vi "progAspicSequence2.vi"(0 "aspic1Data":u32[](array[numeric])=[2863311530, 3149642683, 3435973836, 3722304989, 4008636142, 4294967295, 10, 10, 10, 10, 10, 10, 10, 10, 10, 10, 10, 10, 10, 10, 10, 10, 10, 10, 10, 10, 10, 10, 10, 10, 10, 10] format="%07x", 1 "aspic2Data":u32[](array[numeric])=[2863311530, 3149642683, 3435973836, 3722304989, 4008636142, 4294967295, 10, 10, 10, 10, 10, 10, 10, 10, 10, 10, 10, 10, 10, 10, 10, 10, 10, 10, 10, 10, 10, 10, 10, 10, 10, 10] format="%07x", 2 "aspic3Data":u32[](array[numeric])=[0] format="%07x") -> (9 "error out":errorcluster)   [LabVIEW 2014]
panel:
  in  "aspicmessagetype":u32=21845 format="%x"
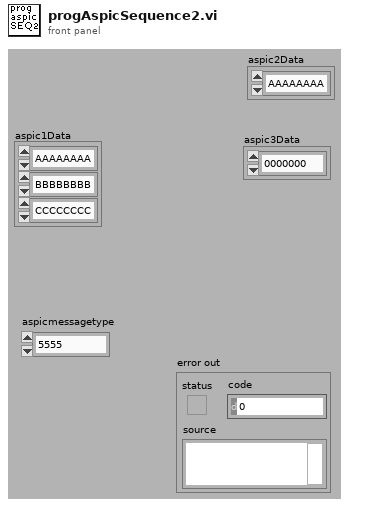
[diagram p1: front panel]
types:
  T1 = enum16{"startTSL", "writeCABAC", "readCABAC", "resetCABAC", "emissionTest", "regRead", "executeASPIC", "resetASPIC", "resetFifo18ASPIC", "resetFifo16ASPIC"}
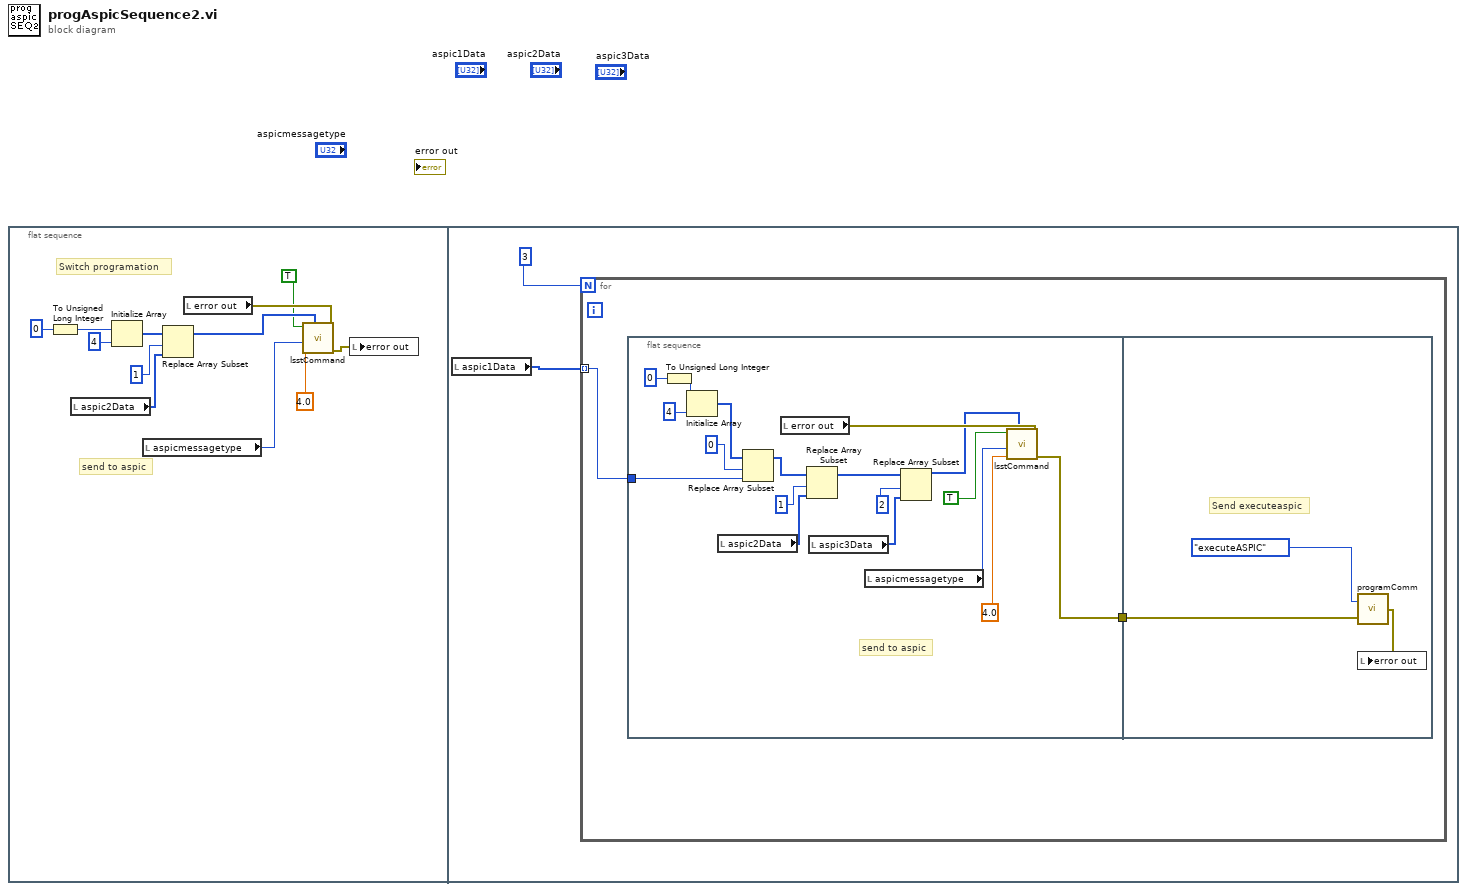
[diagram p0: block diagram]
diagram:
  n1 = flat-sequence {
    frame #0 {
      # "Switch programation"
      # "send to aspic"
      n2 = To Unsigned Long Integer(number=u32 0 ("element")) -> (unsigned 32bit integer=w9:u32)
      n3 = local read "aspic2Data"() -> (w12:u32[])
      n4 = Initialize Array(w9, 4 ("dimension size")) -> (w8:u32[])
      n5 = local read "aspicmessagetype"() -> (w5:u32)
      n6 = Replace Array Subset(array=w8, new element=w12, index=1) -> (w3:u32[])
      n7 = local read "error out"() -> (w4:errorcluster)
      n8 = call "lsstCommand.vi"("error in (no error)"=w4, "data"=w3, "nbitems"=4.0, "messagetype"=w5, "execute"=TRUE) -> ("error out"=w1:errorcluster)  [unwired: 2 in, 4 out]
      n9 = local write "error out"(w1) -> ()
    }
    frame #1 {
      n10 = local read "aspic1Data"() -> (w13:u32[])
      n11 = for {
        N: u8 3 ("aspicitems") -> [_]
        tunnel: w13 -> [w16] mode=indexing
        n12 = flat-sequence {
          tunnel: w16 -> [w22]
          tunnel: [w21] -> w15
          tunnel: w15 -> [w37]
          frame #0 {
            # "send to aspic"
            n13 = To Unsigned Long Integer(number=u32 0 ("element")) -> (unsigned 32bit integer=w28:u32)
            n14 = Initialize Array(w28, 4 ("dimension size")) -> (w27:u32[])
            n15 = local read "aspic2Data"() -> (w25:u32[])
            n16 = Replace Array Subset(array=w27, new element=w22, index=0) -> (w24:u32[])
            n17 = local read "error out"() -> (w34:errorcluster)
            n18 = Replace Array Subset(array=w24, new element=w25, index=1) -> (w19:u32[])
            n19 = local read "aspic3Data"() -> (w17:u32[])
            n20 = local read "aspicmessagetype"() -> (w32:u32)
            n21 = Replace Array Subset(array=w19, new element=w17, index=2) -> (w18:u32[])
            n22 = call "lsstCommand.vi"("error in (no error)"=w34, "data"=w18, "nbitems"=4.0, "messagetype"=w32, "execute"=TRUE) -> ("error out"=w21:errorcluster)  [unwired: 2 in, 4 out]
          }
          frame #1 {
            # "Send executeaspic"
            n23 = call "programComm.vi"("error in (no error)"=w37, "CommSelect"=T1."executeASPIC") -> ("error out"=w35:errorcluster)
            n24 = local write "error out"(w35) -> ()
          }
        }
      }
    }
  }
